vi "Get Height Bounds.vi"(8 "error in (no error)":errorcluster, 11 "Camera in":refnum<class "Camera.lvclass">) -> (0 "error out":errorcluster, 1 "Height Max":i32, 2 "Height Min":i32, 3 "Camera":refnum<class "Camera.lvclass">)   [LabVIEW 2020, in "Camera.lvclass"]
uses:
  Camera.lvclass
  Camera.lvclass/Camera.ctl
  bin/gindustrialcam_32-1.dll
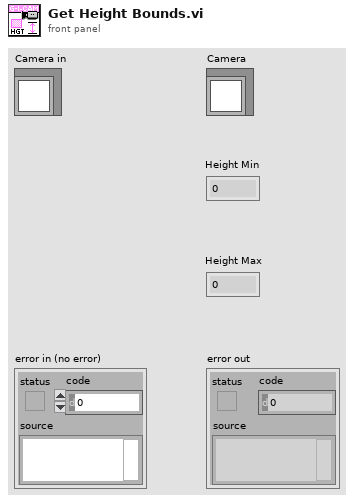
[diagram p1: front panel]
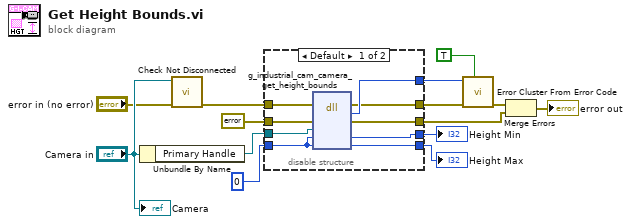
[diagram p0: block diagram]
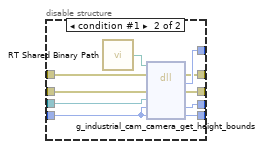
[diagram p2: hidden frame]
diagram:
  n1 = Unbundle By Name("Camera in") -> ("Primary Handle"=w9:refnum<data-value>)
  n2 = call "Check Not Disconnected.vi"("error in (no error)"="error in (no error)", "Camera in"="Camera in") -> ("error out"=w10:errorcluster)  [unwired: 9 in]
  n3 = disable-structure shown="Default" {
    disable-tunnel: [w23 w33] -> w11
    disable-tunnel: w10 -> [w22 w32]
    disable-tunnel: w9 -> [w21 w31]
    disable-tunnel: errorcluster {"status"=FALSE, "code"=0, "source"=""} ("error constant") -> [w20 w30]
    disable-tunnel: [w19 w29] -> w6
    disable-tunnel: [w18 w28] -> w4
    disable-tunnel: [w17 w27] -> w3
    disable-tunnel: [w16 w26] -> w2
    disable-tunnel: 0 ("Value In") -> [w15 w25]
    frame condition #0 (active) {
      n4 = dll-call lib="C:/serenial/lib/g-industrial-camera/LabVIEW/g_industrial_cam/bin/gindustrialcam_*-1.*" fn="g_industrial_cam_camera_get_height_bounds"(error in=w22, "err"=w20, "edvr"=w21, "min"=w15, "max"=w15) -> (error out=w17:errorcluster, "Mg_Error"=w18:i32, "err"=w19:errorcluster, "min"=w23:i32, "max"=w16:i32)  [unwired: 3 in, 1 out]
    }
    frame condition #1 {
      n5 = call "RT Shared Binary Path.vi"() -> ("Path"=w24:path)
      n6 = dll-call lib="C:/serenial/lib/g-industrial-camera/LabVIEW/g_industrial_cam/bin/gindustrialcam_*-1.*" fn="g_industrial_cam_camera_get_height_bounds"(path in=w24, error in=w32, "err"=w30, "edvr"=w31, "min"=w25, "max"=w25) -> (error out=w27:errorcluster, "Mg_Error"=w28:i32, "err"=w29:errorcluster, "min"=w33:i32, "max"=w26:i32)  [unwired: 2 in, 1 out]
    }
  }
  "Height Min" <- w11
  "Height Max" <- w2
  n7 = call <vilib>:"Error Cluster From Error Code.vi"("show call chain? (False)"=TRUE, "error in (no error)"=w3, "error code (0)"=w4) -> ("error out"=w5:errorcluster)  [unwired: 6 in]
  n8 = Merge Errors(w5, w6) -> (→"error out":errorcluster)
  "Camera" <- "Camera in"
